vi "radiansConversion.vi"(9 "encoder":dbl, 10 "setpoint":dbl) -> (0 "encoder (rads)":dbl, 1 "error":dbl, 2 "setpoint (rads)":dbl)   [LabVIEW 2019]
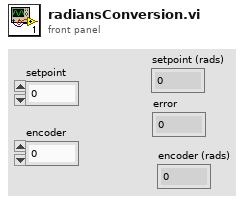
[diagram p1: front panel]
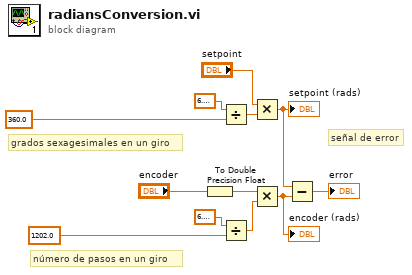
[diagram p0: block diagram]
diagram:
  # "señal de error"
  # "número de pasos en un giro"
  # "grados sexagesimales en un giro"
  n1 = To Double Precision Float(number="encoder") -> (double precision float=w9:dbl)
  n2 = Divide(x=6.283185307179586, y=360.0) -> (x/y=w7:dbl)
  n3 = Divide(x=6.283185307179586, y=1202.0 ("x")) -> (x/y=w10:dbl)
  n4 = Multiply(x="setpoint", y=w7) -> (x*y=w3:dbl)
  "setpoint (rads)" <- w3
  n5 = Multiply(x=w9, y=w10) -> (x*y=w4:dbl)
  "encoder (rads)" <- w4
  n6 = Subtract(x=w3, y=w4) -> (x-y=→"error":dbl)
